vi "HTML Report Table Cell.vi"(4 "vertical align (default)":T2, 5 "pixel size (default)":cluster{"height":i32, "width":i32}, 6 "align (default)":T1, 7 "cell span (1,1)":cluster{"row":i32, "col":i32}={"row"=1, "col"=1}, 8 "nowrap (F)":bool, 9 "cell type (data cell)":enum16{"data cell", "header cell"}(ring), 10 "cell contents":string, 11 "table cells in":string) -> (3 "table cells out":string)   [LabVIEW 2020, in "NI_ReportGenerationCore.lvlib"]
doc: "Constructs tags for an HTML table data or header cell <TD,TR> with the specified cell content."
uses:
  <vilib>/Utility/NIReport.llb/NI_ReportGenerationCore.lvlib
  <vilib>/Utility/NIReport.llb/HTML Report Vertical Cell Alignment.ctl
  <vilib>/Utility/NIReport.llb/HTML Report Text Alignment.ctl
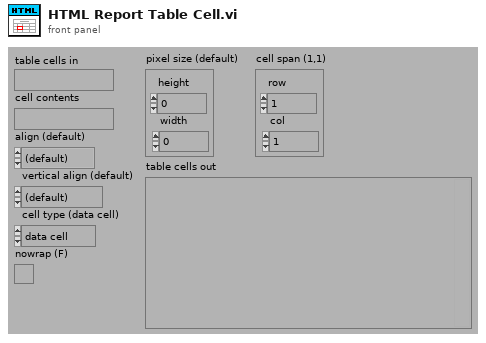
[diagram p1: front panel]
types:
  T1 = typedef "NI_ReportGenerationCore.lvlib/HTML Report Text Alignment.ctl" = enum16{"(default)", "LEFT", "CENTER", "RIGHT"}
  T2 = typedef "NI_ReportGenerationCore.lvlib/HTML Report Vertical Cell Alignment.ctl" = enum16{"(default)", "TOP", "MIDDLE", "BOTTOM"}
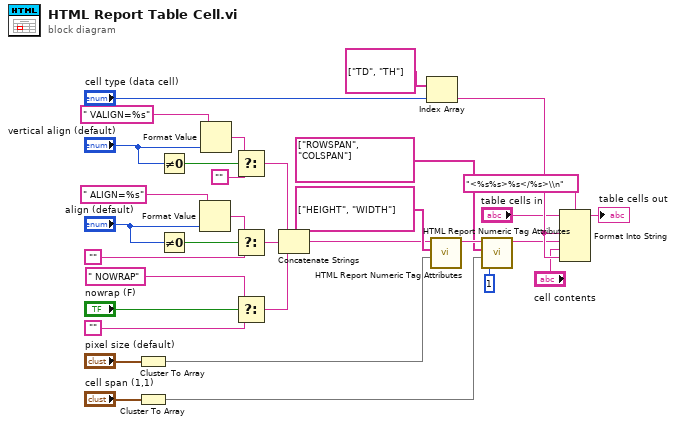
[diagram p0: block diagram]
diagram:
  n1 = Cluster To Array(cluster="pixel size (default)") -> (array=w21:i32[])
  n2 = Cluster To Array(cluster="cell span (1,1)") -> (array=w19:i32[])
  n3 = Not Equal To 0?(x="vertical align (default)") -> (x != 0?=w26:bool)
  n4 = Not Equal To 0?(x="align (default)") -> (x != 0?=w31:bool)
  n5 = Format Value(format string=" ALIGN=%s", value (0)="align (default)") -> (output string=w30:string)  [unwired: 1 out]
  n6 = Format Value(format string=" VALIGN=%s", value (0)="vertical align (default)") -> (output string=w27:string)  [unwired: 1 out]
  n7 = Select(t=w27, s=w26, f="" ("Empty String Constant")) -> (s? t:f=w4:string)
  n8 = Select(t=w30, s=w31, f="" ("Empty String Constant")) -> (s? t:f=w3:string)
  n9 = Select(t=" NOWRAP" ("format string"), s="nowrap (F)", f="" ("Empty String Constant")) -> (s? t:f=w2:string)
  n10 = Concatenate Strings(w4, w3, w2) -> (w1:string)
  n11 = Index Array(array=string[] ["TD", "TH"] ("Labels"), index="cell type (data cell)") -> (element=w12:string)
  n12 = call <vilib>:"HTML Report Numeric Tag Attributes.vi"("values"=w21, "labels"=string[] ["HEIGHT", "WIDTH"] ("Labels"), "tag attributes in"=w1) -> ("tag attributes out"=w18:string)  [unwired: 4 out]
  n13 = call <vilib>:"HTML Report Numeric Tag Attributes.vi"("default value (0)"=1, "values"=w19, "labels"=string[] ["ROWSPAN", "COLSPAN"] ("Labels"), "tag attributes in"=w18) -> ("tag attributes out"=w11:string)  [unwired: 3 out]
  n14 = Format Into String(format string="<%s%s>%s</%s>\\n", initial string="table cells in", w12, w11, "cell contents", w12) -> (resulting string=→"table cells out":string)  [unwired: 1 in, 1 out]
